vi "8164B Lan test.vi"() -> ()   [LabVIEW 2018]
uses:
  KeySight 8164B/KeySight 8164B LAN InstrLib/typedefs/KeySight 8164B APMode.ctl
  KeySight 8164B/KeySight 8164B LAN InstrLib/typedefs/KeySight 8164B Power Unit.ctl
  KeySight 8164B/KeySight 8164B LAN InstrLib.lvlib
panel:
  in  "APMode":T1
  in  "Power Set Point":dbl=-60.0 format="%#_13g"
  in  "stop":bool
  out "Power":dbl format="%#_6p, dBm"
  in  "Att 3, dB":dbl=60.0 format="%#_13g, dB"
  in  "Att 1, dB":dbl=40.0 format="%#_13g, dB"
  in  "Enable":bool
  in  "WaveLength, nm":dbl=1550.0 format="%#_13g, nm"
  out "Slots Info":string[](array[string])
  out "Info":string
  out "error out":errorcluster
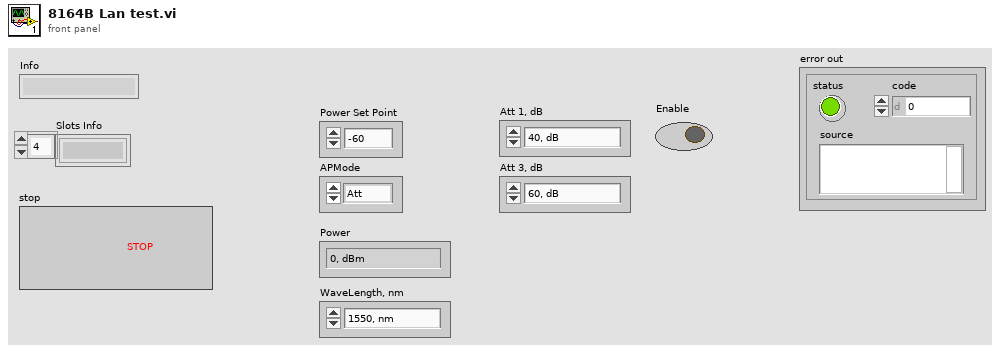
[diagram p1: front panel]
types:
  T1 = typedef "KeySight 8164B LAN InstrLib.lvlib/KeySight 8164B APMode.ctl" = enum16{"Att", "Pset"}
  T2 = typedef "KeySight 8164B LAN InstrLib.lvlib/KeySight 8164B Power Unit.ctl" = enum16{"dBm", "Watt"}
  T3 = typedef "KeySight 8164B LAN InstrLib.lvlib/KeySight 8164B control.ctl" = cluster{"Connection ID":refnum<k5>, "Connected":bool, "Info":string, "Slots Info":string[]}
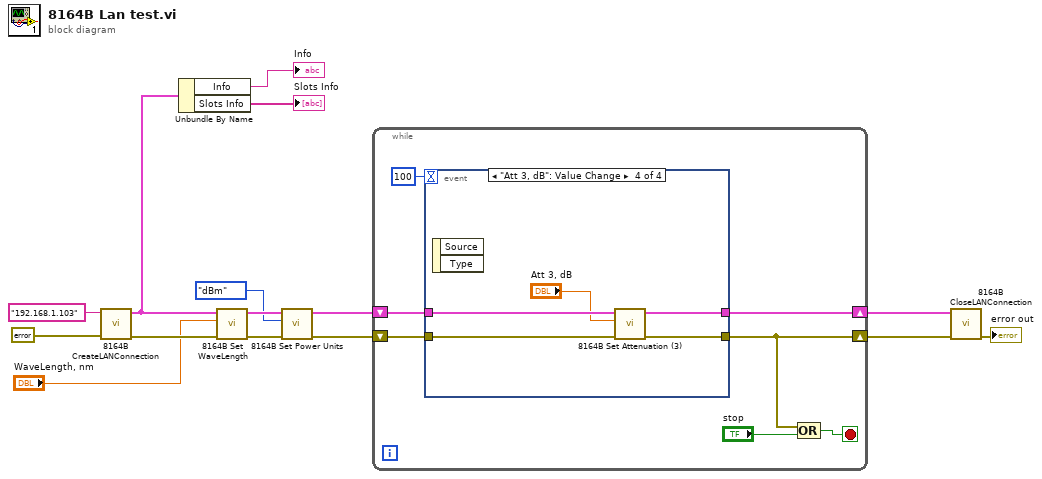
[diagram p0: block diagram]
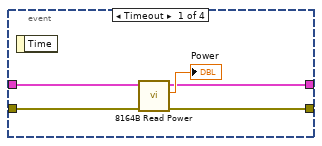
[diagram p2: hidden frame]
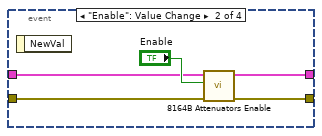
[diagram p3: hidden frame]
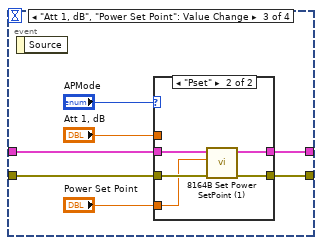
[diagram p4: hidden frame]
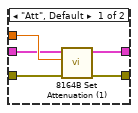
[diagram p5: hidden frame]
diagram:
  n1 = call "8164B CreateLANConnection.vi"("error in"=errorcluster {"status"=FALSE, "code"=0, "source"=""}, "IP address"="192.168.1.103" ("address")) -> ("error out"=w9:errorcluster, "KeySight 8164B control out"=w10:T3)  [unwired: 8 in]
  n2 = Unbundle By Name(w10) -> ("Info"=→"Info":string, "Slots Info"=→"Slots Info":string[])
  n3 = call "8164B Set WaveLength.vi"("error in"=w9, "WaveLength, nm"="WaveLength, nm", "KeySight 8164B control in"=w10) -> ("error out"=w6:errorcluster, "KeySight 8164B control out"=w7:T3)  [unwired: 7 in]
  n4 = call "8164B Set Power Units.vi"("error in"=w6, "Power Unit"=KeySight_8164B_Power_Unit."dBm", "KeySight 8164B control in"=w7) -> ("error out"=w3:errorcluster, "KeySight 8164B control out"=w4:T3)  [unwired: 7 in]
  n5 = while {
    shift-right: [w18] -> w2
    shift-left: w4 -> [w20]
    shift-right: [w16] -> w1
    shift-left: w3 -> [w19]
    stop <- w21 stop-if-true
    n6 = event shown="[3] \"Att 3, dB\": Value Change" {
      selector: _ -> [_ _ _ _]
      dyn-events: _ -> [_ _ _ _]
      timeout: 100 -> [_ _ _ _]
      tunnel: w20 -> [w25 w31 w38 w54]
      tunnel: w19 -> [w26 w30 w36 w53]
      tunnel: [w24 w29 w34 w51] -> w18
      tunnel: [w23 w28 w35 w50] -> w16
      event Timeout {
        n7 = event-data() -> ()  [unwired: 1 in, 1 out]
        n8 = call "8164B Read Power.vi"("error in"=w26, "KeySight 8164B control in"=w25) -> ("error out"=w23:errorcluster, "Power"=→"Power":dbl, "KeySight 8164B control out"=w24:T3)  [unwired: 7 in]
      }
      event "Enable": Value Change {
        n9 = event-data() -> ()  [unwired: 1 in, 1 out]
        n10 = call "8164B Attenuators Enable.vi"("error in"=w30, "Enable"="Enable", "KeySight 8164B control in"=w31) -> ("error out"=w28:errorcluster, "KeySight 8164B control out"=w29:T3)  [unwired: 7 in]
      }
      event "Att 1, dB", "Power Set Point": Value Change {
        n11 = event-data() -> ()  [unwired: 1 in, 1 out]
        n12 = case shown="\"Pset\"" "APMode" {
          tunnel: "Att 1, dB" -> [w44 _]
          tunnel: w38 -> [w43 w49]
          tunnel: w36 -> [w42 w48]
          tunnel: [w41 w46] -> w35
          tunnel: [w40 w47] -> w34
          tunnel: "Power Set Point" -> [_ w45]
          frame "Att", Default {
            n13 = call "8164B Set Attenuation (1).vi"("error in"=w42, "Att 1, dB"=w44, "KeySight 8164B control in"=w43) -> ("error out"=w41:errorcluster, "KeySight 8164B control out"=w40:T3)  [unwired: 7 in]
          }
          frame "Pset" {
            n14 = call "8164B Set Power SetPoint (1).vi"("error in"=w48, "Power Set Point"=w45, "KeySight 8164B control in"=w49) -> ("error out"=w46:errorcluster, "KeySight 8164B control out"=w47:T3)  [unwired: 7 in]
          }
        }
      }
      event "Att 3, dB": Value Change {
        n15 = event-data() -> ()  [unwired: 1 in, 2 out]
        n16 = call "8164B Set Attenuation (3).vi"("error in"=w53, "Att 3, dB"="Att 3, dB", "KeySight 8164B control in"=w54) -> ("error out"=w50:errorcluster, "KeySight 8164B control out"=w51:T3)  [unwired: 7 in]
      }
    }
    n17 = Compound Arithmetic op=OR(w16, "stop") -> (w21:bool)
  }
  n18 = call "8164B CloseLANConnection.vi"("error in"=w1, "KeySight 8164B control"=w2) -> ("error out"=→"error out":errorcluster)  [unwired: 9 in]
